vi "Test_Connection_2.vi"() -> ()   [LabVIEW 2024]
uses:
  <vilib>/LabVIEW Open Source Project/MQTT Control Packets/Control Packets/CONNECT/ConnectFlags -- cluster.ctl
  <vilib>/LabVIEW Open Source Project/MQTT Control Packets/Control Packets/CONNACK/Connect Return Code -- enum.ctl
  <vilib>/LabVIEW Open Source Project/MQTT Client/Client class/Client.lvclass/Client.ctl
  <vilib>/LabVIEW Open Source Project/MQTT Connection/MQTT_Base/Base Class/MQTT_Base.lvclass/MQTT_Base.ctl
  <vilib>/LabVIEW Open Source Project/MQTT Secured TCP Connection/Connection.SecuredTCP/Connection.TCP-TLS.lvclass
  C:/Program Files (x86)/National Instruments/LabVIEW 2024/vi.lib/LabVIEW Open Source Project/Connection/Connection/Connection.lvclass
  <vilib>/LabVIEW Open Source Project/MQTT Client/Client class/Client.lvclass
  C:/Program Files (x86)/National Instruments/LabVIEW 2024/vi.lib/LabVIEW Open Source Project/MQTT Connection/MQTT_Base/Base Class/MQTT_Base.lvclass
  <vilib>/LabVIEW Open Source Project/MQTT Control Packets/Control Packets/PUBLISH/PUBLISH.lvclass
  <vilib>/LabVIEW Open Source Project/MQTT Connection/MQTT_Base/Base Class/MQTT_Base.lvclass
  <vilib>/LabVIEW Open Source Project/MQTT Control Packets/Control Packets/CONNECT/CONNECT.lvclass
  <vilib>/LabVIEW Open Source Project/MQTT Control Packets/Control Packets/CONNACK/CONNACK.lvclass
panel:
  in  "Hostname":string="ce06b4f8ae4542a08357c542c4882795.s1.eu.hivemq.cloud"
  out "Auth Client?":bool=TRUE
  in  "ID (empty:generate new)":string="CustomerAdmin"
  out "Ready for SSL":bool=TRUE
  in  "address (localhost)":string="ce06b4f8ae4542a08357c542c4882795.s1.eu.hivemq.cloud"
  in  "Client X.509 Certificate":path=path "C:/Users/viasl/Desktop/Skole/IIA3220/IIA3220/TestCerts/mqtt-client-cert.crt"
  in  "Client Private Key":path=path "C:/Users/viasl/Desktop/Skole/IIA3220/IIA3220/TestCerts/mqtt-client-key.pem"
  in  "password":string="CustomerAdmin1"
  in  "Server X.509 Certificate":path=path "C:/Users/viasl/Desktop/Skole/IIA3220/IIA3220/TestCerts/isrgrootx1.pem"
  out "Return Code":T1=enum."Server Unavailable"
  in  "Connect Flags":T2={"Reserved"=FALSE, "Clean Session"=TRUE, "Will Flag"=FALSE, "Will QoS 1"=FALSE, "Will QoS 2"=FALSE, "Will Retain"=FALSE, "Password Flag"=FALSE, "User Name Flag"=FALSE}
  in  "Payload":T3={"Will Topic"="", "Will Message"="", "Username"="CustomerClient", "Password"="CustomerClient1"}
  in  "Message":string="commands/topic"
  in  "Connection":bool=TRUE
  in  "Stop Client":bool
  out "Published":bool
  out "last error":errorcluster={"status"=TRUE, "code"=1, "source"="Add Private Key To TLS Configuration in Connection.TCP-TLS.lvclass:onConnection.vi:590001->Connection_GOSPL.lvlib:Connection.lvclass:Connect.vi:3060004->MQTT Client.lvlib:Client.lvclass:Connect to Server.vi:7180001->Test_Connection_2.vi"}
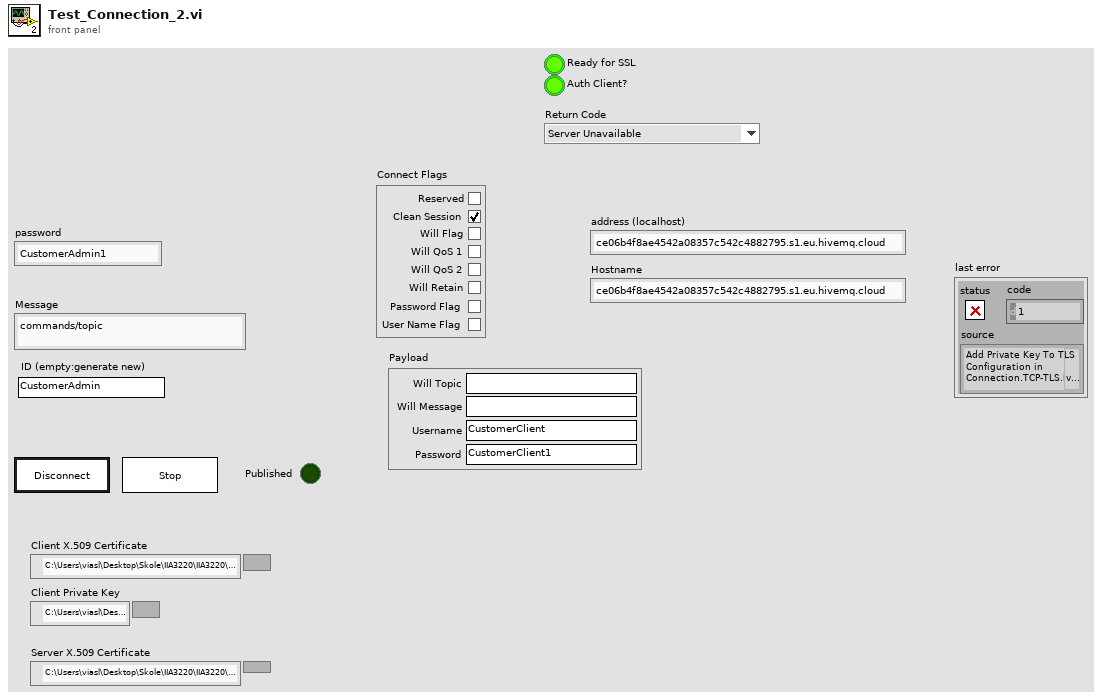
[diagram p1: front panel]
types:
  T1 = typedef "MQTT_Control_Packets.lvlib/CONNACK.lvclass/Connect Return Code -- enum.ctl" = enum16{"Connection accepted", "Unacceptable protocol version", "Identifier Rejected", "Server Unavailable", "Bad Username or Password", "Not Authorized"}
  T2 = typedef "MQTT_Control_Packets.lvlib/CONNECT.lvclass/ConnectFlags -- cluster.ctl" = cluster{"Reserved":bool, "Clean Session":bool, "Will Flag":bool, "Will QoS 1":bool, "Will QoS 2":bool, "Will Retain":bool, "Password Flag":bool, "User Name Flag":bool}
  T3 = cluster{"Will Topic":string, "Will Message":string, "Username":string, "Password":string}
  T4 = typedef "MQTT Client.lvlib/Client.lvclass/Public Events -- cluster.ctl" = cluster{"Connection Status":refnum<user-event>, "Connected":refnum<user-event>, "Application Message":refnum<user-event>}
  T5 = typedef "MQTT Base.lvlib/MQTT_Base.lvclass/Public Events -- cluster.ctl" = cluster{"Stop Event":refnum<user-event>, "Error Event":refnum<user-event>, "Inbound Message":refnum<user-event>}
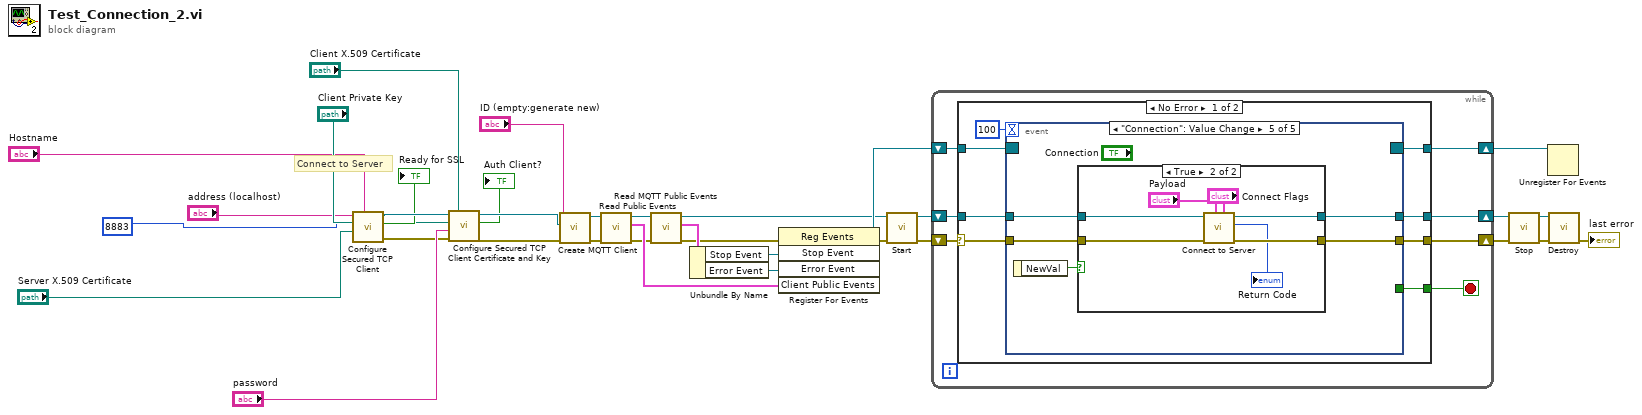
[diagram p0: block diagram]
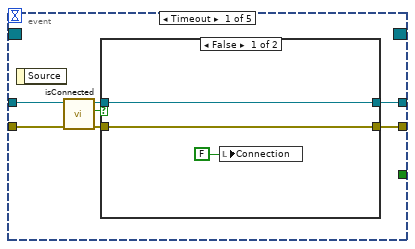
[diagram p2: hidden frame]
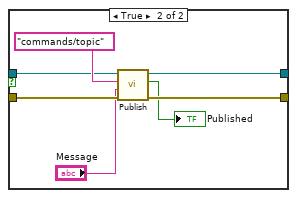
[diagram p3: hidden frame]
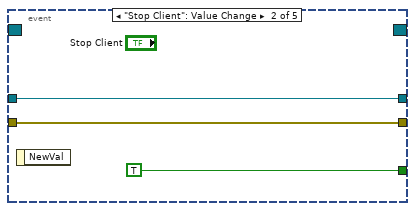
[diagram p4: hidden frame]
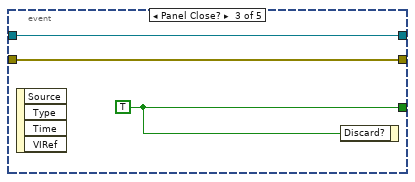
[diagram p5: hidden frame]
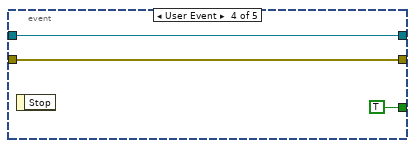
[diagram p6: hidden frame]
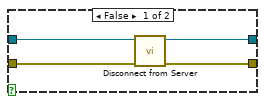
[diagram p7: hidden frame]
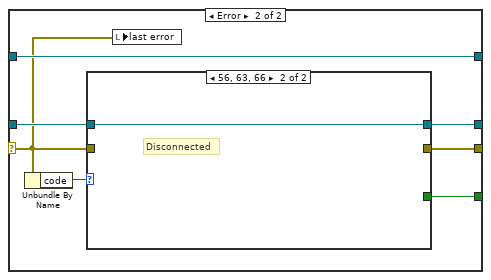
[diagram p8: hidden frame]
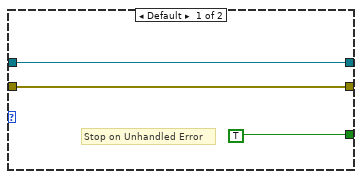
[diagram p9: hidden frame]
diagram:
  # "Connect to Server"
  n1 = call <vilib>:"Configure Secured TCP Client.vi"("Hostname"="Hostname", "Server X.509 Certificate"="Server X.509 Certificate", "remote port (443)"=u16 8883 ("remote port (80)"), "address (localhost)"="address (localhost)") -> ("error out"=w5:errorcluster, "Ready for SSL"=→"Ready for SSL":bool, "Secured TCP Connection"=w14:refnum<class "Connection.TCP-TLS.lvclass">)  [unwired: 5 in]
  n2 = call <vilib>:"Configure Secured TCP Client Certificate and Key.vi"("Client X.509 Certificate"="Client X.509 Certificate", "error in (no error)"=w5, "password"="password", "Client Private Key"="Client Private Key", "Connection.TCP-TLS in"=w14) -> ("error out"=w10:errorcluster, "Auth Client?"=→"Auth Client?":bool, "Connection.TCP-TLS out"=w12:refnum<class "Connection.TCP-TLS.lvclass">)  [unwired: 4 in]
  n3 = call <vilib>:"Create MQTT Client.vi"("error in (no error)"=w10, "Connection Configuration"=w12, "ID (empty:generate new)"="ID (empty:generate new)") -> ("error out"=w17:errorcluster, "Client out"=w15:refnum<class "Client.lvclass">)  [unwired: 7 in]
  n4 = call <vilib>:"Read Public Events.vi"("error in (no error)"=w17, "Client in"=w15) -> ("error out"=w18:errorcluster, "Client Public Events"=w20:T4, "Client out"=w16:refnum<class "Client.lvclass">)  [unwired: 7 in]
  n5 = call <vilib>:"Read MQTT Public Events.vi"("error in (no error)"=w18, "MQTT_Base in"=w16) -> ("error out"=w19:errorcluster, "MQTT Public Events"=w27:T5, "MQTT_Base out"=w22:refnum<class "Client.lvclass">)  [unwired: 7 in]
  n6 = Unbundle By Name(w27) -> ("Stop Event"=w25:refnum<user-event>, "Error Event"=w26:refnum<user-event>)
  n7 = register-events(error in=w19, w25, w26, w20) -> (reference out=w23:refnum<event-registration>, error out=w21:errorcluster)  [unwired: 1 in]
  n8 = call <vilib>:"Start.vi"("error in (no error)"=w21, "MQTT_Base in"=w22) -> ("error out"=w33:errorcluster, "MQTT_Base out"=w32:refnum<class "Client.lvclass">)  [unwired: 7 in, 1 out]
  n9 = while {
    shift-right: [w40] -> w24
    shift-left: w23 -> [w41]
    shift-right: [w37] -> w29
    shift-left: w32 -> [w38]
    shift-right: [w39] -> w31
    shift-left: w33 -> [w35]
    stop <- w36 stop-if-true
    n10 = case shown="No Error" w35 {
      selector: w35 -> [w42 w92]
      tunnel: w41 -> [w49 w98]
      tunnel: [w48 w98] -> w40
      tunnel: [w47 w94] -> w39
      tunnel: w38 -> [w45 w96]
      tunnel: [w44 w95] -> w37
      tunnel: [w43 w93] -> w36
      frame No Error {
        n11 = event shown="[4] \"Connection\": Value Change" {
          selector: w49 -> [_ _ _ _ _]
          dyn-events: [_ _ _ _ _] -> w48
          timeout: 100 -> [_ _ _ _ _]
          tunnel: w42 -> [w52 w68 w70 w75 w76]
          tunnel: [w55 w68 w70 w75 w77] -> w47
          tunnel: [_ TRUE w72 TRUE _] -> w43
          tunnel: w45 -> [w54 w69 w71 w73 w80]
          tunnel: [w56 w69 w71 w73 w78] -> w44
          event Timeout {
            n12 = event-data() -> ()  [unwired: 1 in, 1 out]
            n13 = call <vilib>:"isConnected.vi"("error in (no error)"=w52, "Client in"=w54) -> ("error out"=w51:errorcluster, "connected"=w50:bool, "Client out"=w53:refnum<class "Client.lvclass">)  [unwired: 7 in]
            n14 = case shown="False" w50 {
              tunnel: [w59 w65] -> w56
              tunnel: [w58 w64] -> w55
              tunnel: w53 -> [w59 w62]
              tunnel: w51 -> [w58 w61]
              frame False {
                n15 = local write "Connection"(FALSE ("Connection")) -> ()
              }
              frame True {
                n16 = call <vilib>:"Publish.vi"("error in (no error)"=w61, "Payload"="Message", "Topic Name (empty: Payload name)"="commands/topic", "Client in"=w62) -> ("error out"=w64:errorcluster, "Published"=→"Published":bool, "Client out"=w65:refnum<class "Client.lvclass">)  [unwired: 5 in]
              }
            }
          }
          event "Stop Client": Value Change {
            n17 = event-data() -> ()  [unwired: 1 in, 1 out]
          }
          event Panel Close? {
            w72 = TRUE
            n18 = event-data() -> ()  [unwired: 1 in, 4 out]
            n19 = event-data("Discard?"=w72) -> ()  [unwired: 1 in, 1 out]
          }
          event User Event {
            n20 = event-data() -> ()  [unwired: 1 in, 1 out]
          }
          event "Connection": Value Change {
            n21 = event-data() -> ("NewVal"=w79:bool)  [unwired: 1 in]
            n22 = case shown="True" w79 {
              tunnel: w80 -> [w84 w91]
              tunnel: [w83 w88] -> w78
              tunnel: [w82 w89] -> w77
              tunnel: w76 -> [w81 w90]
              frame False {
                n23 = call <vilib>:"Disconnect from Server.vi"("error in (no error)"=w81, "Client in"=w84) -> ("error out"=w82:errorcluster, "Client out"=w83:refnum<class "Client.lvclass">)  [unwired: 7 in, 1 out]
              }
              frame True {
                n24 = call <vilib>:"Connect to Server.vi"("Connect Flags"="Connect Flags", "Payload"="Payload", "error in (no error)"=w90, "Client in"=w91) -> ("error out"=w89:errorcluster, "Return Code"=→"Return Code":T1, "Client out"=w88:refnum<class "Client.lvclass">)  [unwired: 4 in, 1 out]
              }
            }
          }
        }
      }
      frame Error {
        n25 = Unbundle By Name(w92) -> ("code"=w97:i32)
        n26 = case shown="56, 63, 66" w97 {
          tunnel: w96 -> [w101 w102]
          tunnel: [w101 w102] -> w95
          tunnel: w92 -> [w100 _]
          tunnel: [w100 _] -> w94
          tunnel: [TRUE _] -> w93
          frame Default {
            # "Stop on Unhandled Error"
          }
          frame 56, 63, 66 {
            # "Disconnected"
          }
        }
        n27 = local write "last error"(w92) -> ()
      }
    }
  }
  n28 = call <vilib>:"Stop.vi"("error in (no error)"=w31, "MQTT_Base in"=w29) -> ("error out"=w30:errorcluster, "MQTT_Base out"=w28:refnum<class "Client.lvclass">)  [unwired: 7 in, 1 out]
  n29 = Unregister For Events(event registration refnum=w24) -> ()  [unwired: 1 in, 1 out]
  n30 = call <vilib>:"Destroy.vi"("error in (no error)"=w30, "MQTT_Base in"=w28) -> ("error out"=→"last error":errorcluster)  [unwired: 8 in, 1 out]
